vi "Read Encoders.vi"(9 "Reset Encoders":bool, 11 "Encoder":string="My Counter RefNum") -> (2 "Counts":i32)   [LabVIEW 2014]
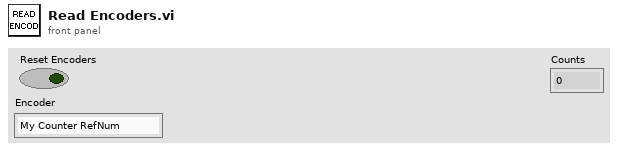
[diagram p1: front panel]
types:
  T1 = typedef "WPI_CounterDevRef.ctl" = cluster{"DevStatus":errorcluster, "CntIndex":T2}
  T2 = typedef "FPGA_CounterCtrSystemIndex.ctl" = enum8{"Ctr 0", "Ctr 1", "Ctr 2", "Ctr 3", "Ctr 4", "Ctr 5", "Ctr 6", "Ctr 7", "Invalid"}
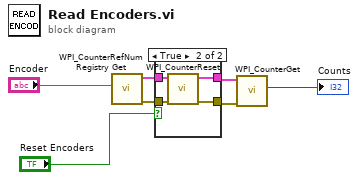
[diagram p0: block diagram]
diagram:
  n1 = call <vilib>:"WPI_CounterRefNum Registry Get.vi"("refnum name"="Encoder") -> ("error out"=w5:errorcluster, "CounterDevRef"=w4:T1)  [unwired: 9 in]
  n2 = case shown="True" "Reset Encoders" {
    tunnel: [w9 w13] -> w7
    tunnel: [w8 w12] -> w6
    tunnel: w4 -> [w9 w11]
    tunnel: w5 -> [w8 w10]
    frame False {
    }
    frame True {
      n3 = call <vilib>:"WPI_CounterReset.vi"("error in (no error)"=w10, "CounterDevRef in"=w11) -> ("error out"=w12:errorcluster, "CounterDevRef out"=w13:T1)  [unwired: 8 in]
    }
  }
  n4 = call <vilib>:"WPI_CounterGet.vi"("error in (no error)"=w6, "CounterDevRef in"=w7) -> ("Value"=→"Counts":i32)  [unwired: 4 in, 5 out]
